vi "lab2_usrp_packet_transceiver2.vi"() -> ()   [LabVIEW 2014]
uses:
  <vilib>/addons/Modulation/Digital/General/MT Generate Bits (Galois, PN Order).vi
  <vilib>/addons/Modulation/Analog/support/mod_Set Error Source.vi
  <vilib>/addons/Modulation/Digital/Support/Common/Validators/mod_Generate Bits Validate.vi
  var_stop.vi
  <vilib>/addons/Modulation/Digital/Support/Common/Validators/mod_Generate Filter Coefficients Validate.vi
  <vilib>/addons/Modulation/Digital/General/subVIs/mod_Generate Filter Coefficients.vi
  <vilib>/measure/maspectr.llb/FFT Power Spectrum and PSD for 1 Chan (CDB).vi
  <vilib>/addons/Modulation/Digital/General/MT Apply Matched Filter (Generic).vi
  <vilib>/addons/Modulation/Digital/General/MT Align to Ideal Symbols (Generic).vi
  <instrlib>/niUSRP/niUSRP Fetch Rx Data (CDB Cluster).vi
  <instrlib>/niUSRP/niUSRP Write Tx Data (CDB Cluster).vi
  <vilib>/addons/Modulation/Digital/General/subVIs/mod_Generate Bits PN Sequence.vi
  <vilib>/addons/Modulation/Digital/General/MT Apply Pulse Shaping Filter (Generic).vi
  <vilib>/addons/Modulation/niDMT.lvlib
  <vilib>/measure/NI_MAPro.lvlib
panel:
  in  "Keep sending":bool
  in  "millisecond multiple":u32=150
  out "Numeric 2":i32
  out "Numeric":i32
  out "x = y?":bool
  in  "Ratio of  redundant":i32=5
  out "ser":dbl
  out "received symbols":dbl
  out "error symbols":i32
  in  "random bits length":i32=50000
  in  "packet bits":i32[](array[numeric])
  out "RX Constellation Map (uneq)":cdb[](graph)
  in  "Transmit power (db)":dbl
  out "ber":dbl
  out "received bits":i32
  out "error bits":i32
  in  "random bits":i8[](array[numeric])
  out "found?":bool
  out "# elements in queue":i32
  out "Spectrum monitor":cluster{"f0":dbl, "df":dbl, "magnitude":dbl[]}(graph)={"f0"=-0.49993781867926873, "df"=0.00012436264146250465, "magnitude"=[]}
  out "RX Constellation Map":cdb[](graph)
  out "valid?":bool
  in  "Gray code?":bool
  in  "Modulation":enum16{"PSK", "QAM"}(ring)=enum."QAM"
  out "Rx String":string
  out "packet len":u32
  in  "Send (deprecated)":bool
  in  "filter length (symbols)":i32=8
  in  "filter parameter":dbl=0.5 format="%.2f"
  in  "pulse shaping filter (none)":T1(ring)=enum."Raised Cosine"
  in  "M-PSK (4)":i32=16 caption="M-ARY"
  in  "samples per symbol (16)":i32=4
  out "packet bits length":i32
  in  "number of samples":i64=40000
  out "RX coerced gain":dbl format="%#_6f"
  out "RX coerced carrier frequency":dbl=915000000.0 format="%#_6p"
  out "RX coerced IQ rate":dbl=4000000.0 format="%#_6p"
  in  "RX active antenna":string="RX2"
  in  "RX gain":dbl format="%#_6f"
  in  "RX device names":refnum<k15>="192.168.10.2"
  out "TX coerced gain":dbl format="%#_6f"
  out "TX coerced carrier frequency":dbl=915000000.0 format="%#_6p"
  out "coerced IQ rate":dbl=4000000.0 format="%#_6p"
  in  "TX device names":refnum<k15>="192.168.10.2"
  in  "TX gain":dbl format="%#_6f"
  in  "carrier frequency":dbl=915000000.0 format="%#_6p"
  in  "IQ rate":dbl=800000.0 format="%#_6p"
  in  "stop":bool
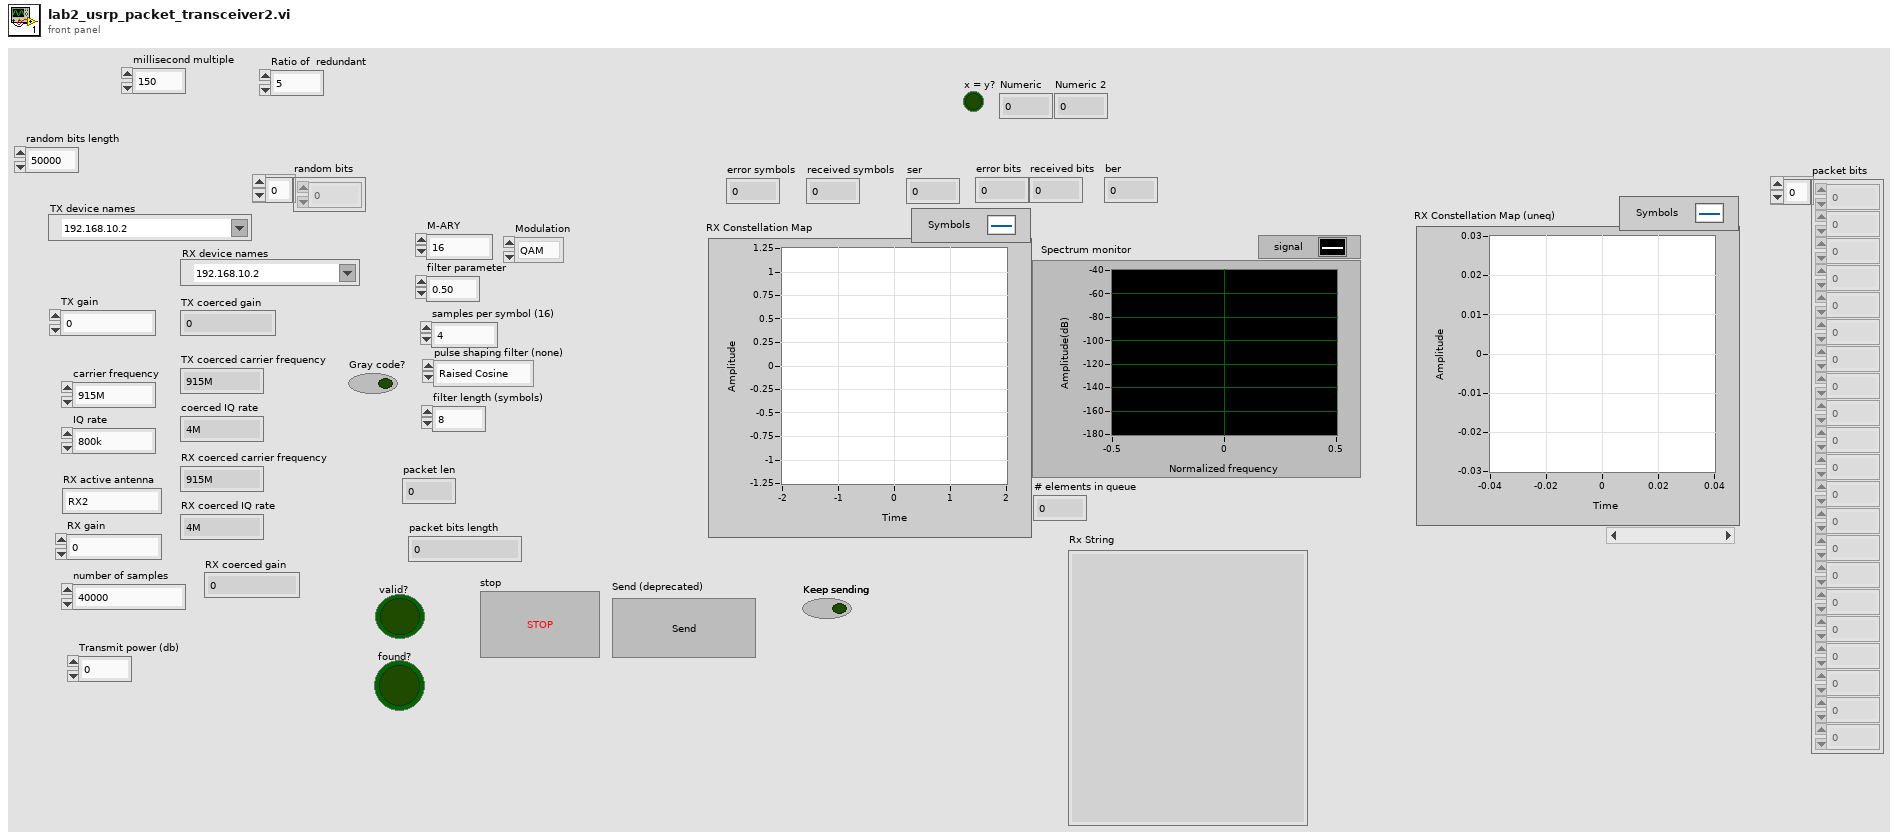
[diagram p1: front panel]
types:
  T1 = enum16{"none", "Raised Cosine", "Root Raised Cos", "Gaussian"}
  T2 = enum16{"FSK", "PSK", "QAM", "MSK", "PAM", "ASK", "CPM"}
  T3 = cluster{"samples per symbol (16)":i32, "symbol map":cdb[], "index map":u32[]}
  T4 = cluster{"samples per symbol (16)":i32, "symbol map":cdb[], i32[]}
  T5 = typedef "niAMT.lvlib/Complex Data Waveform.ctl" = cluster{"t0":dbl, "dt":dbl, "Y":cdb[]}
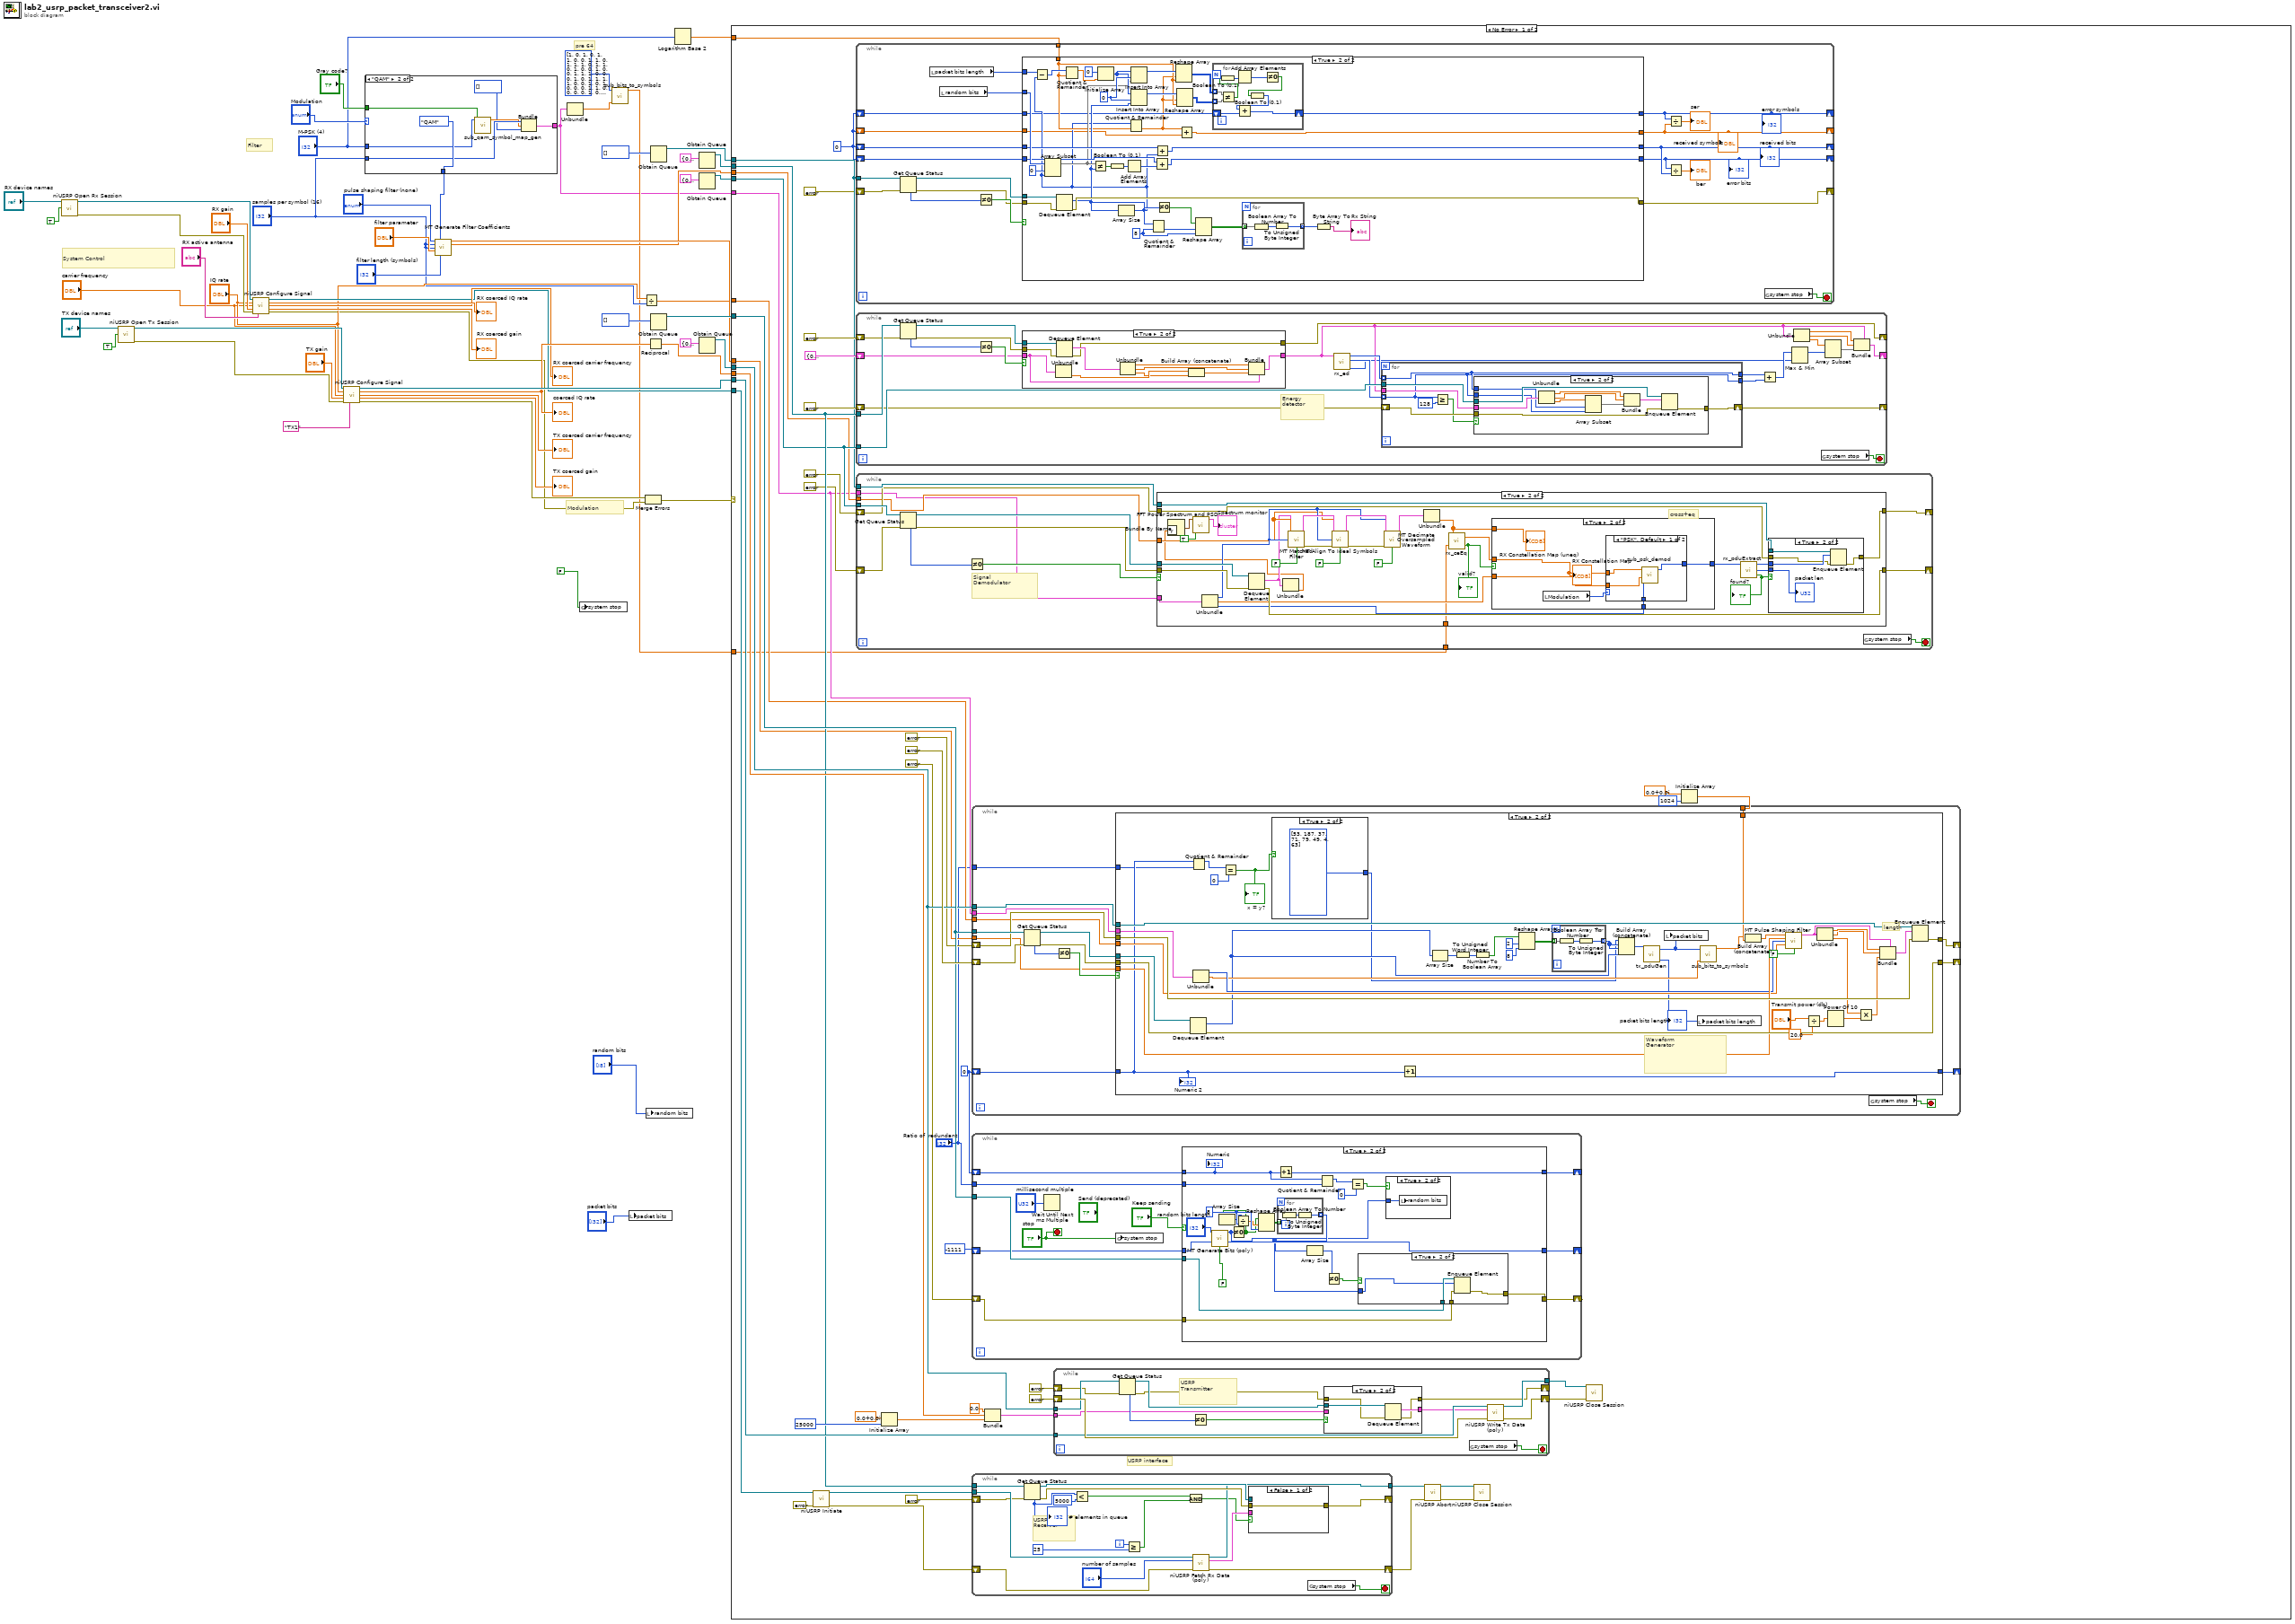
[diagram p0: block diagram]
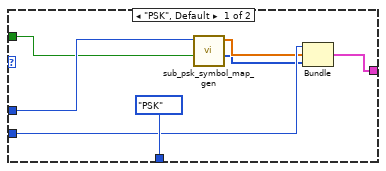
[diagram p2: hidden frame]
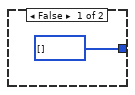
[diagram p5: hidden frame]
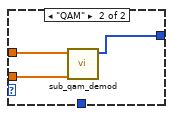
[diagram p6: hidden frame]
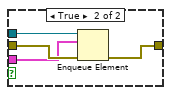
[diagram p10: hidden frame]
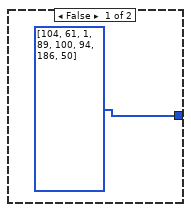
[diagram p13: hidden frame]
diagram:
  # "pre 64"
  # "Modulation"
  # "Filter"
  # "System Control"
  n1 = call <instrlib>:"niUSRP Open Rx Session.vi"("device names"="RX device names", "reset"=TRUE) -> ("session handle out"=w41:refnum<k15>, "error out"=w40:errorcluster)  [unwired: 12 in]
  n2 = call <instrlib>:"niUSRP Open Tx Session.vi"("device names"="TX device names", "reset"=TRUE) -> ("session handle out"=w54:refnum<k15>, "error out"=w53:errorcluster)  [unwired: 12 in]
  n3 = call <instrlib>:"niUSRP Configure Signal.vi"("session handle"=w41, "IQ rate"="IQ rate", "carrier frequency"="carrier frequency", "gain"="RX gain", "error in (no error)"=w40, "active antenna"="RX active antenna") -> ("session handle out"=w32:refnum<k15>, "coerced IQ rate"=→"RX coerced IQ rate":dbl, "coerced carrier frequency"=→"RX coerced carrier frequency":dbl, "coerced gain"=→"RX coerced gain":dbl, "error out"=w16:errorcluster)  [unwired: 5 in]
  n4 = call <instrlib>:"niUSRP Configure Signal.vi"("session handle"=w54, "IQ rate"="IQ rate", "carrier frequency"="carrier frequency", "gain"="TX gain", "error in (no error)"=w53, "active antenna"="TX1") -> ("session handle out"=w45:refnum<k15>, "coerced IQ rate"=w43:dbl, "coerced carrier frequency"=→"TX coerced carrier frequency":dbl, "coerced gain"=→"TX coerced gain":dbl, "error out"=w17:errorcluster)  [unwired: 5 in]
  "coerced IQ rate" <- w43
  n5 = case shown="\"QAM\"" "Modulation" {
    tunnel: [T2."PSK" ("modulation type") T2."QAM" ("modulation type")] -> w11
    tunnel: "M-PSK (4)" -> [w61 w67]
    tunnel: "Gray code?" -> [w60 w68]
    tunnel: "samples per symbol (16)" -> [w59 w66]
    tunnel: [w56 w63] -> w5
    frame "PSK", Default {
      n6 = call "sub_psk_symbol_map_gen.vi"("Gray code?"=w60, "M-PSK"=w61) -> ("index map"=w57:u32[], "symbol map"=w58:cdb[])  [unwired: 8 in]
      n7 = Bundle("samples per symbol (16)"=w59, "symbol map"=w58, "index map"=w57) -> (w56:T3)  [unwired: 1 in]
    }
    frame "QAM" {
      n8 = call "sub_qam_symbol_map_gen.vi"("Gray code?"=w68, "M-QAM"=w67) -> ("symbol map"=w65:cdb[])  [unwired: 9 in]
      n9 = Bundle("samples per symbol (16)"=w66, "symbol map"=w65, i32[] []) -> (w63:T4)  [unwired: 1 in]
    }
  }
  n10 = call <vilib>:"MT Generate Filter Coefficients.vi"("pulse shaping filter (none)"="pulse shaping filter (none)", "modulation type"=w11, "pulse shaping samples per symbol (16)"="samples per symbol (16)", "matched samples per symbol (16)"="samples per symbol (16)", "filter parameter"="filter parameter", "filter length (symbols)"="filter length (symbols)") -> ("pulse shaping filter coefficients"=w22:dbl[], "matched filter coefficients"=w20:dbl[])  [unwired: 7 in, 1 out]
  n11 = Unbundle(w5) -> ("symbol map"=w7:cdb[])  [unwired: 2 out]
  n12 = global write "var_stop.vi" "system stop"(FALSE) -> ()
  n13 = call "sub_bits_to_symbols.vi"("symbol map"=w7, "bits"=i16[] [1, 0, 1, 0, 1, 1, 0, 0, 1, 1, 0, 1, 1, 1, 0, 1, 1, 0, 1, 0, 0, 1, 0, 0, 1, 1, 1, 0, 0, 0, 1, 0, 1, 1, 1, 1, 0, 0, 1, 0, 1, 0, 0, 0, 1, 1, 0, 0, 0, 0, 1, 0, 0, 0, 0, 0, 1, 1, 1, 1, 1, 1, 0, 0] ("preamble(64) 2")) -> ("symbols"=w6:cdb[])  [unwired: 9 in]
  n14 = local write "packet bits"("packet bits") -> ()
  n15 = Divide(x="IQ rate", y="samples per symbol (16)") -> (x/y=w21:dbl)
  n16 = Merge Errors(w17, w16) -> (w15:errorcluster)
  n17 = local write "random bits"("random bits") -> ()
  n18 = Reciprocal(x=w43) -> (1/x=w42:dbl)
  n19 = Obtain Queue(element data type=i8[] [] ("output bit stream")) -> (queue out=w27:refnum<queue>)  [unwired: 4 in, 2 out]
  n20 = Obtain Queue(element data type=i16[] []) -> (queue out=w55:refnum<queue>)  [unwired: 4 in, 2 out]
  n21 = Logarithm Base 2(1:"M-PSK (4)") -> (0:w2:dbl)
  n22 = Obtain Queue(element data type=cluster{"t0":dbl, "dt":dbl, "Y":cdb[]} {"t0"=0.0, "dt"=0.0, "Y"=[]} ("data")) -> (queue out=w31:refnum<queue>)  [unwired: 4 in, 2 out]
  n23 = Obtain Queue(element data type=cluster{"t0":dbl, "dt":dbl, "Y":cdb[]} {"t0"=0.0, "dt"=0.0, "Y"=[]} ("data")) -> (queue out=w28:refnum<queue>)  [unwired: 4 in, 2 out]
  n24 = Obtain Queue(element data type=cluster{"t0":dbl, "dt":dbl, "Y":cdb[]} {"t0"=0.0, "dt"=1.0, "Y"=[]} ("data")) -> (queue out=w46:refnum<queue>)  [unwired: 4 in, 2 out]
  n25 = case shown="No Error" w15 {
    tunnel: w55 -> [w115 _]
    tunnel: w46 -> [w110 _]
    tunnel: w45 -> [w111 _]
    tunnel: w42 -> [w104 _]
    tunnel: w32 -> [w99 _]
    tunnel: w31 -> [w93 _]
    tunnel: w28 -> [w89 _]
    tunnel: w27 -> [w87 _]
    tunnel: w5 -> [w81 _]
    tunnel: w22 -> [w84 _]
    tunnel: w21 -> [w83 _]
    tunnel: w20 -> [w82 _]
    tunnel: w6 -> [w75 _]
    tunnel: w2 -> [w73 _]
    frame No Error {
      w71 = 0
      w72 = 0
      # "USRP interface"
      n26 = call <instrlib>:"niUSRP Initiate.vi"("session handle"=w99, "error in (no error)"=errorcluster {"status"=FALSE, "code"=0, "source"=""}) -> ("session handle out"=w98:refnum<k15>, "error out"=w97:errorcluster)  [unwired: 12 in]
      n27 = while {
        tunnel: w87 -> [w137]
        shift-right: [w130] -> _
        shift-left: errorcluster {"status"=FALSE, "code"=0, "source"=""} ("error out") -> [w136]
        shift-right: [w125] -> _
        shift-left: w72 -> [w128]
        shift-right: [w126] -> _
        shift-left: w72 -> [w127]
        tunnel: w73 -> [w122]
        shift-right: [w119] -> _
        shift-left: w72 -> [w121]
        shift-right: [w118] -> _
        shift-left: w72 -> [w120]
        stop <- w135 stop-if-true
        n28 = Get Queue Status(queue=w137, error in (no error)=w136) -> (queue out=w132:refnum<queue>, error out=w131:errorcluster, # elements in queue=w134:i32)  [unwired: 1 in, 5 out]
        n29 = local read "packet bits length"() -> (w123:i32)
        n30 = local read "random bits"() -> (w129:i8[])
        n31 = Not Equal To 0?(x=w134) -> (x != 0?=w133:bool)
        n32 = case shown="True" w133 {
          tunnel: w132 -> [_ w179]
          tunnel: w131 -> [w142 w178]
          tunnel: [w142 w173] -> w130
          tunnel: w129 -> [_ w170]
          tunnel: w128 -> [w141 w166]
          tunnel: [w141 w165] -> w125
          tunnel: [w140 w163] -> w126
          tunnel: w127 -> [w140 w164]
          tunnel: w123 -> [_ w155]
          tunnel: w122 -> [_ w151]
          tunnel: w121 -> [w139 w147]
          tunnel: [w139 w146] -> w119
          tunnel: w120 -> [w138 w145]
          tunnel: [w138 w143] -> w118
          frame False {
          }
          frame True {
            w159 = 0
            w176 = 8 ("y")
            n33 = Dequeue Element(queue=w179, error in (no error)=w178) -> (element=w156:i8[], error out=w173:errorcluster)  [unwired: 1 in, 2 out]
            n34 = Array Size(array=w156) -> (size(s)=w150:i32)
            n35 = Subtract(x=w155, y=w150) -> (x-y=w154:i32)
            n36 = Array Subset(array=w170, index=0, length=w150) -> (w157:i8[])
            n37 = Quotient & Remainder(x=w154, y=w151) -> (x-y*floor(x/y)=w160:dbl)  [unwired: 1 out]
            n38 = Not Equal?(x=w157, y=w156) -> (x != y?=w169:bool[])
            n39 = Initialize Array(0, w160) -> (w158:i32[])
            n40 = Boolean To (0,1)(Boolean=w169) -> (0, 1=w168:i16[])
            n41 = Add Array Elements(numeric array=w168) -> (sum=w167:i16)
            n42 = Quotient & Remainder(x=w150, y=w151) -> (floor(x/y)=w144:dbl)  [unwired: 1 out]
            n43 = Insert Into Array(array=w158, index=w159, new element=w157) -> (w153:i32[])
            n44 = Insert Into Array(array=w158, index=w159, new element=w156) -> (w152:i32[])
            n45 = Quotient & Remainder(x=w150, y=w176) -> (floor(x/y)=w175:i32)  [unwired: 1 out]
            n46 = Add(x=w166, y=w167) -> (x+y=w165:i32)
            n47 = Add(x=w164, y=w150) -> (x+y=w163:i32)
            n48 = Not Equal To 0?(x=w156) -> (x != 0?=w177:bool[])
            n49 = Reshape Array(w153, w144, w151) -> (w149:i32[][])
            n50 = Reshape Array(w152, w144, w151) -> (w148:i32[][])
            n51 = Add(x=w144, y=w145) -> (x+y=w143:dbl)
            n52 = Reshape Array(w177, w175, w176) -> (w174:bool[][])
            n53 = for {
              tunnel: w149 -> [w187] mode=indexing
              tunnel: w148 -> [w188] mode=indexing
              shift-right: [w183] -> w146
              shift-left: w147 -> [w182]
              n54 = Not Equal?(x=w187, y=w188) -> (x != y?=w186:bool[])
              n55 = Boolean To (0,1)(Boolean=w186) -> (0, 1=w185:i16[])
              n56 = Add Array Elements(numeric array=w185) -> (sum=w184:i16)
              n57 = Not Equal To 0?(x=w184) -> (x != 0?=w181:bool)
              n58 = Boolean To (0,1)(Boolean=w181) -> (0, 1=w180:i16)
              n59 = Add(x=w180, y=w182) -> (x+y=w183:i32)
            }
            n60 = for {
              tunnel: w174 -> [w191] mode=indexing
              tunnel: [w190] -> w172 mode=indexing
              n61 = Boolean Array To Number(Boolean array=w191) -> (number=w189:u32)
              n62 = To Unsigned Byte Integer(number=w189) -> (unsigned 8bit integer=w190:u8)
            }
            n63 = Byte Array To String(unsigned byte array=w172) -> (string=→"Rx String":string)
          }
        }
        "error bits" <- w125
        "received bits" <- w126
        "error symbols" <- w119
        "received symbols" <- w118
        n64 = Divide(x=w119, y=w118) -> (x/y=→"ser":dbl)
        n65 = Divide(x=w125, y=w126) -> (x/y=→"ber":dbl)
        n66 = global read "var_stop.vi" "system stop"() -> (w135:bool)
      }
      n67 = while {
        tunnel: w93 -> [w284]
        shift-right: [w277] -> _
        shift-left: errorcluster {"status"=FALSE, "code"=0, "source"=""} ("error out") -> [w283]
        shift-right: [w263] -> _
        shift-left: cluster{"t0":dbl, "dt":dbl, "Y":cdb[]} {"t0"=0.0, "dt"=0.0, "Y"=[]} ("data") -> [w278]
        tunnel: w89 -> [w276]
        shift-right: [w275] -> _
        shift-left: errorcluster {"status"=FALSE, "code"=0, "source"=""} ("error out") -> [w274]
        stop <- w273 stop-if-true
        # "Energy\ndetector"
        n68 = Get Queue Status(queue=w284, error in (no error)=w283) -> (queue out=w279:refnum<queue>, error out=w280:errorcluster, # elements in queue=w282:i32)  [unwired: 1 in, 5 out]
        n69 = Not Equal To 0?(x=w282) -> (x != 0?=w281:bool)
        n70 = case shown="True" w281 {
          tunnel: w280 -> [w306 w317]
          tunnel: w279 -> [_ w316]
          tunnel: w278 -> [w305 w311]
          tunnel: [w306 w308] -> w277
          tunnel: [w305 w307] -> w270
          frame False {
          }
          frame True {
            n71 = Unbundle(w311) -> ("Y"=w314:cdb[])  [unwired: 2 out]
            n72 = Dequeue Element(queue=w316, error in (no error)=w317) -> (element=w315:cluster{"t0":dbl, "dt":dbl, "Y":cdb[]}, error out=w308:errorcluster)  [unwired: 1 in, 2 out]
            n73 = Unbundle(w315) -> ("t0"=w310:dbl, "dt"=w309:dbl, "Y"=w313:cdb[])
            n74 = Build Array (concatenate)(w314, w313) -> (w312:cdb[])
            n75 = Bundle(cluster=w311, "t0"=w310, "dt"=w309, "Y"=w312) -> (w307:cluster{"t0":dbl, "dt":dbl, "Y":cdb[]})
          }
        }
        n76 = call "rx_ed.vi"("Wavefrom"=w270) -> ("first pulse"=w260:i32, "length"=w271:i32[], "start index"=w272:i32[])  [unwired: 8 in]
        n77 = for {
          tunnel: w276 -> [w292]
          tunnel: w270 -> [w289]
          shift-right: [w291] -> w275
          shift-left: w274 -> [w290]
          tunnel: w272 -> [w288] mode=indexing
          tunnel: w271 -> [w287] mode=indexing
          tunnel: [w288] -> w266
          tunnel: [w287] -> w265
          n78 = Greater Or Equal?(x=w287, y=128) -> (x >= y?=w285:bool)
          n79 = case shown="True" w285 {
            tunnel: w292 -> [_ w304]
            tunnel: [w293 w303] -> w291
            tunnel: w290 -> [w293 w302]
            tunnel: w289 -> [_ w301]
            tunnel: w288 -> [_ w295]
            tunnel: w287 -> [_ w294]
            frame False {
            }
            frame True {
              n80 = Unbundle(w301) -> ("t0"=w299:dbl, "dt"=w300:dbl, "Y"=w297:cdb[])
              n81 = Array Subset(array=w297, index=w295, length=w294) -> (w296:cdb[])
              n82 = Bundle("t0"=w299, "dt"=w300, w296) -> (w298:cluster{"t0":dbl, "dt":dbl, cdb[]})  [unwired: 1 in]
              n83 = Enqueue Element(queue=w304, element=w298, error in (no error)=w302) -> (error out=w303:errorcluster)  [unwired: 1 in, 2 out]
            }
          }
        }
        n84 = Add(x=w266, y=w265) -> (x+y=w262:i32)
        n85 = Max & Min(x=w262, y=w260) -> (max(x,y)=w261:i32)  [unwired: 1 out]
        n86 = Unbundle(w270) -> ("t0"=w269:dbl, "dt"=w268:dbl, "Y"=w267:cdb[])
        n87 = global read "var_stop.vi" "system stop"() -> (w273:bool)
        n88 = Array Subset(array=w267, index=w261) -> (w264:cdb[])  [unwired: 1 in]
        n89 = Bundle(cluster=w270, "t0"=w269, "dt"=w268, "Y"=w264) -> (w263:cluster{"t0":dbl, "dt":dbl, "Y":cdb[]})
      }
      n90 = while {
        tunnel: w89 -> [w205]
        shift-right: [w199] -> _
        shift-left: errorcluster {"status"=FALSE, "code"=0, "source"=""} ("error out") -> [w204]
        tunnel: w87 -> [w198]
        shift-right: [w197] -> _
        shift-left: errorcluster {"status"=FALSE, "code"=0, "source"=""} ("error out") -> [w196]
        tunnel: w82 -> [w194]
        tunnel: w81 -> [w193]
        tunnel: w75 -> [w192]
        stop <- w195 stop-if-true
        # "Signal \nDemodulator"
        n91 = Get Queue Status(queue=w205, error in (no error)=w204) -> (queue out=w201:refnum<queue>, error out=w200:errorcluster, # elements in queue=w203:i32)  [unwired: 1 in, 5 out]
        n92 = Not Equal To 0?(x=w203) -> (x != 0?=w202:bool)
        n93 = case shown="True" w202 {
          tunnel: w201 -> [_ w238]
          tunnel: w200 -> [w207 w239]
          tunnel: [w207 w237] -> w199
          tunnel: w198 -> [_ w230]
          tunnel: [w206 w229] -> w197
          tunnel: w196 -> [w206 w228]
          tunnel: w194 -> [_ w217]
          tunnel: w193 -> [_ w221]
          tunnel: w192 -> [_ w213]
          frame False {
          }
          frame True {
            # "cross+eq"
            n94 = Unbundle(w221) -> ("samples per symbol (16)"=w220:i32, "symbol map"=w219:cdb[], "index map"=w218:u32[])
            n95 = Dequeue Element(queue=w238, error in (no error)=w239) -> (element=w212:cluster{"t0":dbl, "dt":dbl, "Y":cdb[]}, error out=w237:errorcluster)  [unwired: 1 in, 2 out]
            n96 = Unbundle(w212) -> ("Y"=w211:cdb[])  [unwired: 2 out]
            n97 = Bundle By Name("Y"=w211) -> (w216:waveform(cdb))  [unwired: 1 in]
            n98 = call-poly <vilib>:"FFT Power Spectrum and PSD.vi"("dB On (F)"=TRUE, "time signal"=w216) -> ("Power Spectrum / PSD"=→"Spectrum monitor":cluster{"f0":dbl, "df":dbl, "magnitude":dbl[]})  [unwired: 6 in, 3 out]
            n99 = call-poly <vilib>:"MT Matched Filter.vi"("input complex waveform"=w212, "matched filter coefficients"=w217, "samples per symbol (16)"=w220, "reset? (T)"=FALSE) -> ("output complex waveform"=w236:T5, "error out"=w235:errorcluster)  [unwired: 10 in]
            n100 = call-poly <vilib>:"MT Align To Ideal Symbols.vi"("input complex waveform"=w236, "matched filter coefficients"=w217, "samples per symbol (16)"=w220, "error in (no error)"=w235, "reset? (T)"=FALSE) -> ("output complex waveform"=w233:T5, "error out"=w234:errorcluster)  [unwired: 8 in, 1 out]
            n101 = call <vilib>:"MT Decimate Oversampled Waveform.vi"("input complex waveform"=w233, "decimation factor"=w220, "error in (no error)"=w234, "reset? (T)"=FALSE) -> ("output complex waveform"=w232:T5)  [unwired: 10 in, 1 out]
            n102 = Unbundle(w232) -> ("Y"=w210:cdb[])  [unwired: 2 out]
            n103 = call "rx_ceEq.vi"("preamble"=w213, "symbols"=w210) -> ("valid?"=w226:bool, "eq symbols"=w227:cdb[])
            "valid?" <- w226
            n104 = case shown="True" w226 {
              tunnel: [i8[] [] ("output bit stream") w244] -> w209
              tunnel: w219 -> [_ w245]
              tunnel: w227 -> [_ w242]
              tunnel: w218 -> [_ w243]
              tunnel: w210 -> [_ w241]
              frame False {
              }
              frame True {
                n105 = local read "Modulation"() -> (w246:enum16{"PSK", "QAM"})
                n106 = case shown="\"PSK\", Default" w246 {
                  tunnel: w242 -> [w250 w253]
                  tunnel: w245 -> [w249 w252]
                  tunnel: [w247 w251] -> w244
                  tunnel: w243 -> [w248 _]
                  frame "PSK", Default {
                    n107 = call "sub_psk_demod.vi"("index map"=w248, "symbol map"=w249, "symbol"=w250) -> ("bitstream"=w247:i16[])  [unwired: 8 in]
                  }
                  frame "QAM" {
                    n108 = call "sub_qam_demod.vi"("symbol map"=w252, "symbol"=w253) -> ("bitstream"=w251:i16[])  [unwired: 9 in]
                  }
                }
                "RX Constellation Map" <- w242
                "RX Constellation Map (uneq)" <- w241
              }
            }
            n109 = call "rx_pduExtract.vi"("output bit stream"=w209) -> ("found?"=w231:bool, "packet len"=w225:u32, "ppdu"=w208:i8[])  [unwired: 2 in]
            "found?" <- w231
            n110 = case shown="True" w231 {
              tunnel: w208 -> [_ w257]
              tunnel: w230 -> [_ w259]
              tunnel: [w254 w258] -> w229
              tunnel: w228 -> [w254 w255]
              tunnel: w225 -> [_ w256]
              frame False {
              }
              frame True {
                n111 = Enqueue Element(queue=w259, element=w257, error in (no error)=w255) -> (error out=w258:errorcluster)  [unwired: 1 in, 2 out]
                "packet len" <- w256
              }
            }
          }
        }
        n112 = global read "var_stop.vi" "system stop"() -> (w195:bool)
      }
      n113 = Initialize Array(cdb 0.0+0.0i, 25000 ("dimension size")) -> (w105:cdb[])
      n114 = while {
        tunnel: w115 -> [w440]
        shift-right: [w438] -> _
        shift-left: errorcluster {"status"=FALSE, "code"=0, "source"=""} ("error out") -> [w439]
        shift-right: [w436] -> _
        shift-left: -1111 -> [w437]
        shift-right: [w433] -> _
        shift-left: w71 -> [w434]
        tunnel: "Ratio of  redundant" -> [w432]
        stop <- "stop" stop-if-true
        n115 = Wait Until Next ms Multiple(millisecond multiple="millisecond multiple") -> ()  [unwired: 1 out]
        n116 = global write "var_stop.vi" "system stop"("stop") -> ()
        n117 = case shown="True" "Keep sending" {
          tunnel: w440 -> [_ w465]
          tunnel: w439 -> [w444 w464]
          tunnel: [w444 w463] -> w438
          tunnel: w437 -> [w443 w460]
          tunnel: [w443 w459] -> w436
          tunnel: w434 -> [w442 w445]
          tunnel: [w442 w450] -> w433
          tunnel: w432 -> [_ w451]
          frame False {
          }
          frame True {
            w457 = 8
            n118 = call-poly <vilib>:"MT Generate Bits (poly).vi"("total bits (128)"="random bits length", "seed in (0xD6BF7DF2)"=w460, "reset? (T)"=FALSE) -> ("output bit stream"=w447:i8[], "seed out"=w459:i32)  [unwired: 10 in, 1 out]
            n119 = Not Equal To 0?(x=w447) -> (x != 0?=w452:bool[])
            n120 = Array Size(array=w452) -> (size(s)=w456:i32)
            n121 = Divide(x=w456, y=w457) -> (x/y=w455:dbl)
            n122 = Reshape Array(w452, w455, w457) -> (w454:bool[][])
            n123 = for {
              tunnel: w454 -> [w470] mode=indexing
              tunnel: [w468] -> w453 mode=indexing
              n124 = Boolean Array To Number(Boolean array=w470) -> (number=w469:u32)
              n125 = To Unsigned Byte Integer(number=w469) -> (unsigned 8bit integer=w468:u8)
            }
            n126 = Increment(x=w445) -> (x+1=w450:i32)
            n127 = Array Size(array=w453) -> (size(s)=w462:i32)
            n128 = Quotient & Remainder(x=w445, y=w451) -> (x-y*floor(x/y)=w446:i32)  [unwired: 1 out]
            n129 = Not Equal To 0?(x=w462) -> (x != 0?=w466:bool)
            n130 = Equal?(x=w446, y=0) -> (x = y?=w448:bool)
            n131 = case shown="True" w466 {
              tunnel: w453 -> [_ w472]
              tunnel: w465 -> [_ w475]
              tunnel: w464 -> [w471 w474]
              tunnel: [w471 w473] -> w463
              frame False {
              }
              frame True {
                n132 = Enqueue Element(queue=w475, element=w472, error in (no error)=w474) -> (error out=w473:errorcluster)  [unwired: 1 in, 2 out]
              }
            }
            n133 = case shown="True" w448 {
              tunnel: w447 -> [_ w467]
              frame False {
              }
              frame True {
                n134 = local write "random bits"(w467) -> ()
              }
            }
            "Numeric" <- w445
          }
        }
      }
      n135 = while {
        tunnel: w98 -> [w336]
        shift-right: [w324] -> w94
        shift-left: w97 -> [w335]
        tunnel: w93 -> [w333]
        shift-right: [w327] -> _
        shift-left: errorcluster {"status"=FALSE, "code"=0, "source"=""} ("error out") -> [w332]
        tunnel: [w325] -> w95
        i -> [w322]
        stop <- w323 stop-if-true
        # "USRP\nReceiver"
        n136 = Get Queue Status(queue=w333, error in (no error)=w332) -> (queue out=w329:refnum<queue>, error out=w328:errorcluster, # elements in queue=w331:i32)  [unwired: 1 in, 5 out]
        "# elements in queue" <- w331
        n137 = Less?(x=w331, y=5000) -> (x < y?=w320:bool)
        n138 = Greater Or Equal?(x=w322, y=25) -> (x >= y?=w319:bool)
        n139 = And(x=w320, y=w319) -> (x .and. y?=w318:bool)
        n140 = call-poly <instrlib>:"niUSRP Fetch Rx Data (poly).vi"("session handle"=w336, "number of samples"="number of samples", "error in (no error)"=w335) -> ("session handle out"=w325:refnum<k15>, "data"=w326:cluster{"t0":dbl, "dt":dbl, "Y":cdb[]}, "error out"=w324:errorcluster)  [unwired: 9 in, 1 out]
        n141 = case shown="False" w318 {
          tunnel: w329 -> [_ w341]
          tunnel: w328 -> [w337 w340]
          tunnel: [w337 w339] -> w327
          tunnel: w326 -> [_ w338]
          frame False {
          }
          frame True {
            n142 = Enqueue Element(queue=w341, element=w338, error in (no error)=w340) -> (error out=w339:errorcluster)  [unwired: 1 in, 2 out]
          }
        }
        n143 = global read "var_stop.vi" "system stop"() -> (w323:bool)
      }
      n144 = Bundle(0.0, w104, w105) -> (w102:cluster{dbl, dbl, cdb[]})  [unwired: 1 in]
      n145 = while {
        shift-right: [w351] -> w114
        shift-left: errorcluster {"status"=FALSE, "code"=0, "source"=""} ("error out") -> [w349]
        tunnel: [w350] -> w113
        tunnel: w111 -> [w348]
        tunnel: w110 -> [w346]
        shift-right: [w344] -> _
        shift-left: errorcluster {"status"=FALSE, "code"=0, "source"=""} ("error out") -> [w345]
        tunnel: w102 -> [w343]
        stop <- w342 stop-if-true
        # "USRP\nTransmitter"
        n146 = Get Queue Status(queue=w346, error in (no error)=w345) -> (queue out=w353:refnum<queue>, error out=w352:errorcluster, # elements in queue=w355:i32)  [unwired: 1 in, 5 out]
        n147 = Not Equal To 0?(x=w355) -> (x != 0?=w354:bool)
        n148 = case shown="True" w354 {
          tunnel: w353 -> [_ w361]
          tunnel: w352 -> [w356 w360]
          tunnel: [w357 w359] -> w347
          tunnel: [w356 w358] -> w344
          tunnel: w343 -> [w357 _]
          frame False {
          }
          frame True {
            n149 = Dequeue Element(queue=w361, error in (no error)=w360) -> (element=w359:cluster{"t0":dbl, "dt":dbl, "Y":cdb[]}, error out=w358:errorcluster)  [unwired: 1 in, 2 out]
          }
        }
        n150 = global read "var_stop.vi" "system stop"() -> (w342:bool)
        n151 = call-poly <instrlib>:"niUSRP Write Tx Data (poly).vi"("session handle"=w348, "data"=w347, "error in (no error)"=w349) -> ("session handle out"=w350:refnum<k15>, "error out"=w351:errorcluster)  [unwired: 11 in]
      }
      n152 = call <instrlib>:"niUSRP Abort.vi"("session handle"=w95, "error in (no error)"=w94) -> ("session handle out"=w101:refnum<k15>, "error out"=w100:errorcluster)  [unwired: 12 in]
      n153 = call <instrlib>:"niUSRP Close Session.vi"("session handle"=w101, "error in (no error)"=w100) -> ()  [unwired: 13 in, 1 out]
      n154 = call <instrlib>:"niUSRP Close Session.vi"("session handle"=w113, "error in (no error)"=w114) -> ()  [unwired: 13 in, 1 out]
      n155 = Initialize Array(cdb 0.0+0.0i, 1024 ("dimension size")) -> (w76:cdb[])
      n156 = while {
        tunnel: w115 -> [w376]
        shift-right: [w373] -> _
        shift-left: errorcluster {"status"=FALSE, "code"=0, "source"=""} ("error out") -> [w379]
        tunnel: w110 -> [w372]
        shift-right: [w371] -> _
        shift-left: errorcluster {"status"=FALSE, "code"=0, "source"=""} ("error out") -> [w370]
        tunnel: w81 -> [w368]
        tunnel: w84 -> [w367]
        tunnel: w83 -> [w366]
        tunnel: w76 -> [w365]
        shift-right: [w363] -> _
        shift-left: w71 -> [w364]
        tunnel: "Ratio of  redundant" -> [w362]
        stop <- w369 stop-if-true
        n157 = Get Queue Status(queue=w376, error in (no error)=w379) -> (queue out=w374:refnum<queue>, error out=w375:errorcluster, # elements in queue=w378:i32)  [unwired: 1 in, 5 out]
        n158 = Not Equal To 0?(x=w378) -> (x != 0?=w377:bool)
        n159 = case shown="True" w377 {
          tunnel: w375 -> [w382 w425]
          tunnel: w374 -> [_ w424]
          tunnel: [w382 w423] -> w373
          tunnel: w372 -> [_ w418]
          tunnel: [w381 w417] -> w371
          tunnel: w370 -> [w381 w416]
          tunnel: w368 -> [_ w414]
          tunnel: w367 -> [_ w413]
          tunnel: w366 -> [_ w412]
          tunnel: w365 -> [_ w402]
          tunnel: w364 -> [w380 w387]
          tunnel: [w380 w389] -> w363
          tunnel: w362 -> [_ w384]
          frame False {
          }
          frame True {
            # "length"
            # "Waveform \nGenerator"
            n160 = Dequeue Element(queue=w424, error in (no error)=w425) -> (element=w399:i16[], error out=w423:errorcluster)  [unwired: 1 in, 2 out]
            n161 = Quotient & Remainder(x=w387, y=w384) -> (x-y*floor(x/y)=w383:i32)  [unwired: 1 out]
            n162 = Unbundle(w414) -> ("samples per symbol (16)"=w408:i32, "symbol map"=w401:cdb[])  [unwired: 1 out]
            n163 = Equal?(x=w383, y=0) -> (x = y?=w385:bool)
            "x = y?" <- w385
            n164 = case shown="True" w385 {
              tunnel: [u8[] [104, 61, 1, 89, 100, 94, 186, 50] ("Array 2") u8[] [53, 187, 37, 71, 79, 49, 4, 63] ("Array 2")] -> w388
              frame False {
              }
              frame True {
              }
            }
            n165 = Increment(x=w387) -> (x+1=w389:i32)
            n166 = Array Size(array=w399) -> (size(s)=w410:i32)
            n167 = To Unsigned Word Integer(number=w410) -> (unsigned 16bit integer=w409:u16)
            n168 = Number To Boolean Array(number=w409) -> (Boolean array=w422:bool[])
            n169 = Reshape Array(w422, 2 ("dimension size"), 8 ("dimension size")) -> (w419:bool[][])
            n170 = for {
              tunnel: w419 -> [w430] mode=indexing
              tunnel: [w428] -> w411 mode=indexing
              n171 = Boolean Array To Number(Boolean array=w430) -> (number=w429:u32)
              n172 = To Unsigned Byte Integer(number=w429) -> (unsigned 8bit integer=w428:u8)
            }
            n173 = Build Array (concatenate)(w388, w411, w411, w399) -> (w415:i16[])
            n174 = call "tx_pduGen.vi"("byte array"=w415) -> ("packet bits length"=w390:i32, "pdu"=w392:i32[])  [unwired: 3 in]
            "packet bits length" <- w390
            n175 = local write "packet bits"(w392) -> ()
            n176 = local write "packet bits length"(w390) -> ()
            n177 = call "sub_bits_to_symbols.vi"("symbol map"=w401, "bits"=w392) -> ("symbols"=w400:cdb[])  [unwired: 9 in]
            n178 = Build Array (concatenate)(w400, w402) -> (w398:cdb[])
            n179 = call-poly <vilib>:"MT Pulse Shaping Filter.vi"("symbols"=w398, "pulse shaping filter coefficients"=w413, "samples per symbol (16)"=w408, "symbol rate (Hz)"=w412, "reset? (T)"=FALSE) -> ("output complex waveform"=w407:T5)  [unwired: 9 in, 1 out]
            n180 = Divide(x="Transmit power (db)", y=20.0) -> (x/y=w395:dbl)
            n181 = Unbundle(w407) -> ("t0"=w406:dbl, "dt"=w405:dbl, "Y"=w394:cdb[])
            n182 = Power Of 10(x=w395) -> (10^x=w393:dbl)
            n183 = Multiply(x=w394, y=w393) -> (x*y=w391:cdb[])
            n184 = Bundle(cluster=w407, "t0"=w406, "dt"=w405, "Y"=w391) -> (w404:T5)
            n185 = Enqueue Element(queue=w418, element=w404, error in (no error)=w416) -> (error out=w417:errorcluster)  [unwired: 1 in, 2 out]
            "Numeric 2" <- w387
          }
        }
        n186 = global read "var_stop.vi" "system stop"() -> (w369:bool)
      }
    }
    frame Error {
    }
  }
